vi "Create Setpoint Profile.vi"() -> ()   [LabVIEW 2012]
panel:
  in  "Distance":dbl
  in  "Times":T1
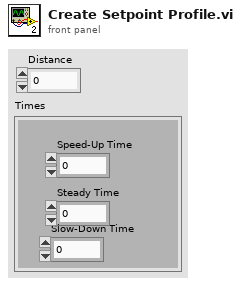
[diagram p1: front panel]
types:
  T1 = cluster{"Speed-Up Time":dbl, "Steady Time":dbl, "Slow-Down Time":dbl}
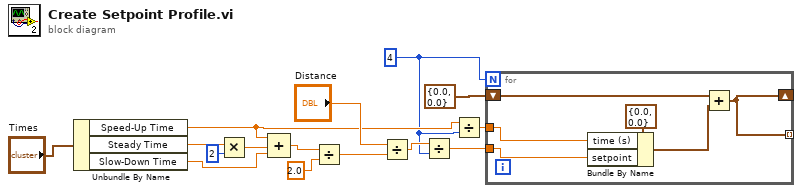
[diagram p0: block diagram]
diagram:
  w2 = 4
  n1 = Unbundle By Name("Times") -> ("Speed-Up Time"=w3:dbl, "Steady Time"=w14:dbl, "Slow-Down Time"=w11:dbl)
  n2 = Multiply(x=w14, y=2) -> (x*y=w12:dbl)
  n3 = Compound Arithmetic op=ADD(w3, w12, w11) -> (w10:dbl)
  n4 = Divide(x=w10, y=2.0) -> (x/y=w8:dbl)
  n5 = Divide(x="Distance", y=w8) -> (x/y=w6:dbl)
  n6 = Divide(x=w6, y=w2) -> (x/y=w5:dbl)
  n7 = Divide(x=w3, y=w2) -> (x/y=w1:dbl)
  n8 = for {
    N: w2 -> [_]
    tunnel: w5 -> [w20]
    shift-right: [w16] -> _
    shift-left: cluster{"time (s)":dbl, "setpoint":dbl} {"time (s)"=0.0, "setpoint"=0.0} -> [w18]
    tunnel: w1 -> [w17]
    tunnel: [w16] -> _ mode=indexing
    n9 = Bundle By Name(cluster=cluster{"time (s)":dbl, "setpoint":dbl} {"time (s)"=0.0, "setpoint"=0.0}, "time (s)"=w17, "setpoint"=w20) -> (w19:cluster{"time (s)":dbl, "setpoint":dbl})
    n10 = Add(x=w18, y=w19) -> (x+y=w16:cluster{"time (s)":dbl, "setpoint":dbl})
  }
